vi "Headers.vi"(8 "error in (no error)":errorcluster, 11 "LabVIEW Web Service Request":refnum<class "Web Request.lvclass">) -> (0 "error out":errorcluster, 3 "LabVIEW Web Service Request out":refnum<class "Web Request.lvclass">)   [LabVIEW 2014]
doc: "Sets all required headers by the SSE connection"
uses:
  <vilib>/wsapi/Web Request.lvclass
  Configuration/Global_Configurations.vi
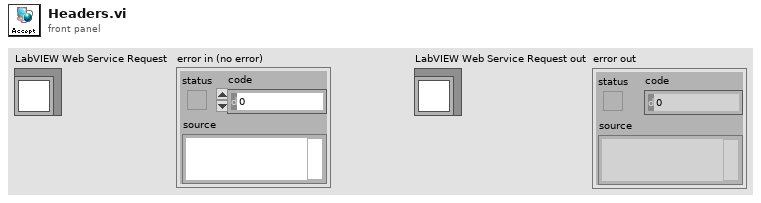
[diagram p1: front panel]
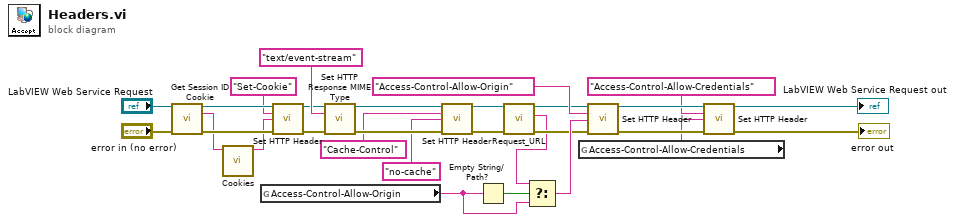
[diagram p0: block diagram]
diagram:
  n1 = call <vilib>:"Get Session ID Cookie.vi"("LabVIEW Web Service Request"="LabVIEW Web Service Request", "error in (no error)"="error in (no error)") -> ("LabVIEW Web Service Request out"=w23:refnum<class "Web Request.lvclass">, "session ID cookie"=w17:string, "error out"=w24:errorcluster)  [unwired: 11 in]
  n2 = call "Cookies.vi"("ID cookie"=w17) -> ("cookie header"=w22:string)  [unwired: 10 in]
  n3 = global read "Global_Configurations.vi" "Access-Control-Allow-Origin"() -> (w9:string)
  n4 = call <vilib>:"Set HTTP Header.vi"("LabVIEW Web Service Request"=w23, "header"="Set-Cookie", "header value"=w22, "error in (no error)"=w24) -> ("LabVIEW Web Service Request out"=w20:refnum<class "Web Request.lvclass">, "error out"=w19:errorcluster)  [unwired: 10 in]
  n5 = call <vilib>:"Set HTTP Response MIME Type.vi"("LabVIEW Web Service Request"=w20, "MIME type (text/html)"="text/event-stream" ("header"), "error in (no error)"=w19) -> ("LabVIEW Web Service Request out"=w29:refnum<class "Web Request.lvclass">, "error out"=w28:errorcluster)  [unwired: 11 in]
  n6 = call <vilib>:"Set HTTP Header.vi"("LabVIEW Web Service Request"=w29, "header"="Cache-Control", "header value"="no-cache", "error in (no error)"=w28) -> ("LabVIEW Web Service Request out"=w5:refnum<class "Web Request.lvclass">, "error out"=w4:errorcluster)  [unwired: 10 in]
  n7 = Empty String/Path?(string/path=w9) -> (empty?=w10:bool)
  n8 = call "Request_URL.vi"("error in (no error)"=w4, "LabVIEW Web Service Request"=w5) -> ("error out"=w2:errorcluster, "Request URL"=w1:string, "LabVIEW Web Service Request out"=w3:refnum<class "Web Request.lvclass">)  [unwired: 7 in]
  n9 = Select(t=w1, s=w10, f=w9) -> (s? t:f=w8:string)
  n10 = global read "Global_Configurations.vi" "Access-Control-Allow-Credentials"() -> (w7:string)
  n11 = call <vilib>:"Set HTTP Header.vi"("LabVIEW Web Service Request"=w3, "header"="Access-Control-Allow-Origin", "header value"=w8, "error in (no error)"=w2) -> ("LabVIEW Web Service Request out"=w15:refnum<class "Web Request.lvclass">, "error out"=w14:errorcluster)  [unwired: 10 in]
  n12 = call <vilib>:"Set HTTP Header.vi"("LabVIEW Web Service Request"=w15, "header"="Access-Control-Allow-Credentials", "header value"=w7, "error in (no error)"=w14) -> ("LabVIEW Web Service Request out"=→"LabVIEW Web Service Request out":refnum<class "Web Request.lvclass">, "error out"=→"error out":errorcluster)  [unwired: 10 in]
